vi "tppathcr.vi"(1 "input":i32) -> (0 "out":string)   [LabVIEW 2015]
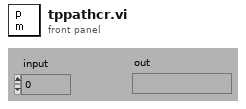
[diagram p1: front panel]
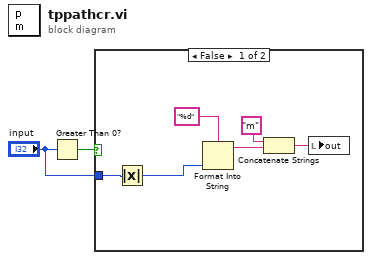
[diagram p0: block diagram]
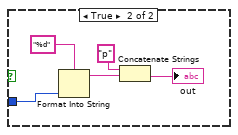
[diagram p2: hidden frame]
diagram:
  n1 = Greater Than 0?(x="input") -> (x > 0?=w2:bool)
  n2 = case shown="False" w2 {
    tunnel: "input" -> [w5 w12]
    frame False {
      n3 = Absolute Value(x=w5) -> (abs(x)=w4:i32)
      n4 = Format Into String(format string="%d", w4) -> (resulting string=w6:string)  [unwired: 2 in, 1 out]
      n5 = Concatenate Strings("m", w6) -> (w3:string)
      n6 = local write "out"(w3) -> ()
    }
    frame True {
      n7 = Format Into String(format string="%d", w12) -> (resulting string=w10:string)  [unwired: 2 in, 1 out]
      n8 = Concatenate Strings("p", w10) -> (→"out":string)
    }
  }
